vi "运维调试_氨氮.vi"() -> ()   [LabVIEW 2016, in "斯坦道氨氮.lvlib"]
uses:
  <vilib>/Utility/miscctls.llb/LVPointTypeDef.ctl
  <vilib>/Utility/config.llb/NI_LVConfig.lvlib
  <vilib>/ptbypt/NI_PtbyPt.lvlib
panel:
  in  "量程参数读取":T1
  in  "模块启用":bool
  in  "串口设置":bool
  in  "公式一键写入":bool
  in  "流程文件路径":path=path "C:/Users/Hsiao/Documents/斯坦道流程文件/流程.xml"
  in  "曲线模型":cluster{"X^2":dbl, "X":dbl, "B":dbl}(xcontrol)
  in  "质控参数设置":bool
  out "字符串":string
  in  "氨氮自动测试量程配置":T2
  out "ADC":sgl
  out "温度2":sgl
  out "温度1":sgl
  out "固件版本号":string
  in  "数组":string[](array[string])
  in  "备用系数写入":bool
  in  "备用系数读取":bool
  in  "参数下拉列表":enum16{"氨氮", "总磷"}(ring)
  in  "量程下拉列表":enum16{"低量程", "高量程"}(ring)
  in  "测量模式下拉列表":enum16{"水样测量", "空白核查", "跨度核查", "标样核查", "加标回收"}(ring)
  in  "公式":cluster{"X^2":dbl, "X":dbl, "b":dbl}
  in  "写公式":bool
  in  "读公式":bool
  in  "返回":bool
  in  "设置":bool
  out "序列号":string="序列号"
  out "氨氮测量数据":T3(xcontrol)
  out "集成报警信息":string
  out "定时启动":bool
  out "总磷总氮运行状态":T4(xcontrol)
  in  "停止":bool
  in  "手动启动":bool
  in  "单步测试":bool
  in  "总磷氨氮调试":u16[](xcontrol)
  out "F3":sgl format="%#.6f"
  out "F2":sgl format="%#.6f"
  out "F1":sgl format="%#.6f"
  out "F0":sgl format="%#.6f"
  out "多列列表框":i32(listbox)
  # "参数设置"
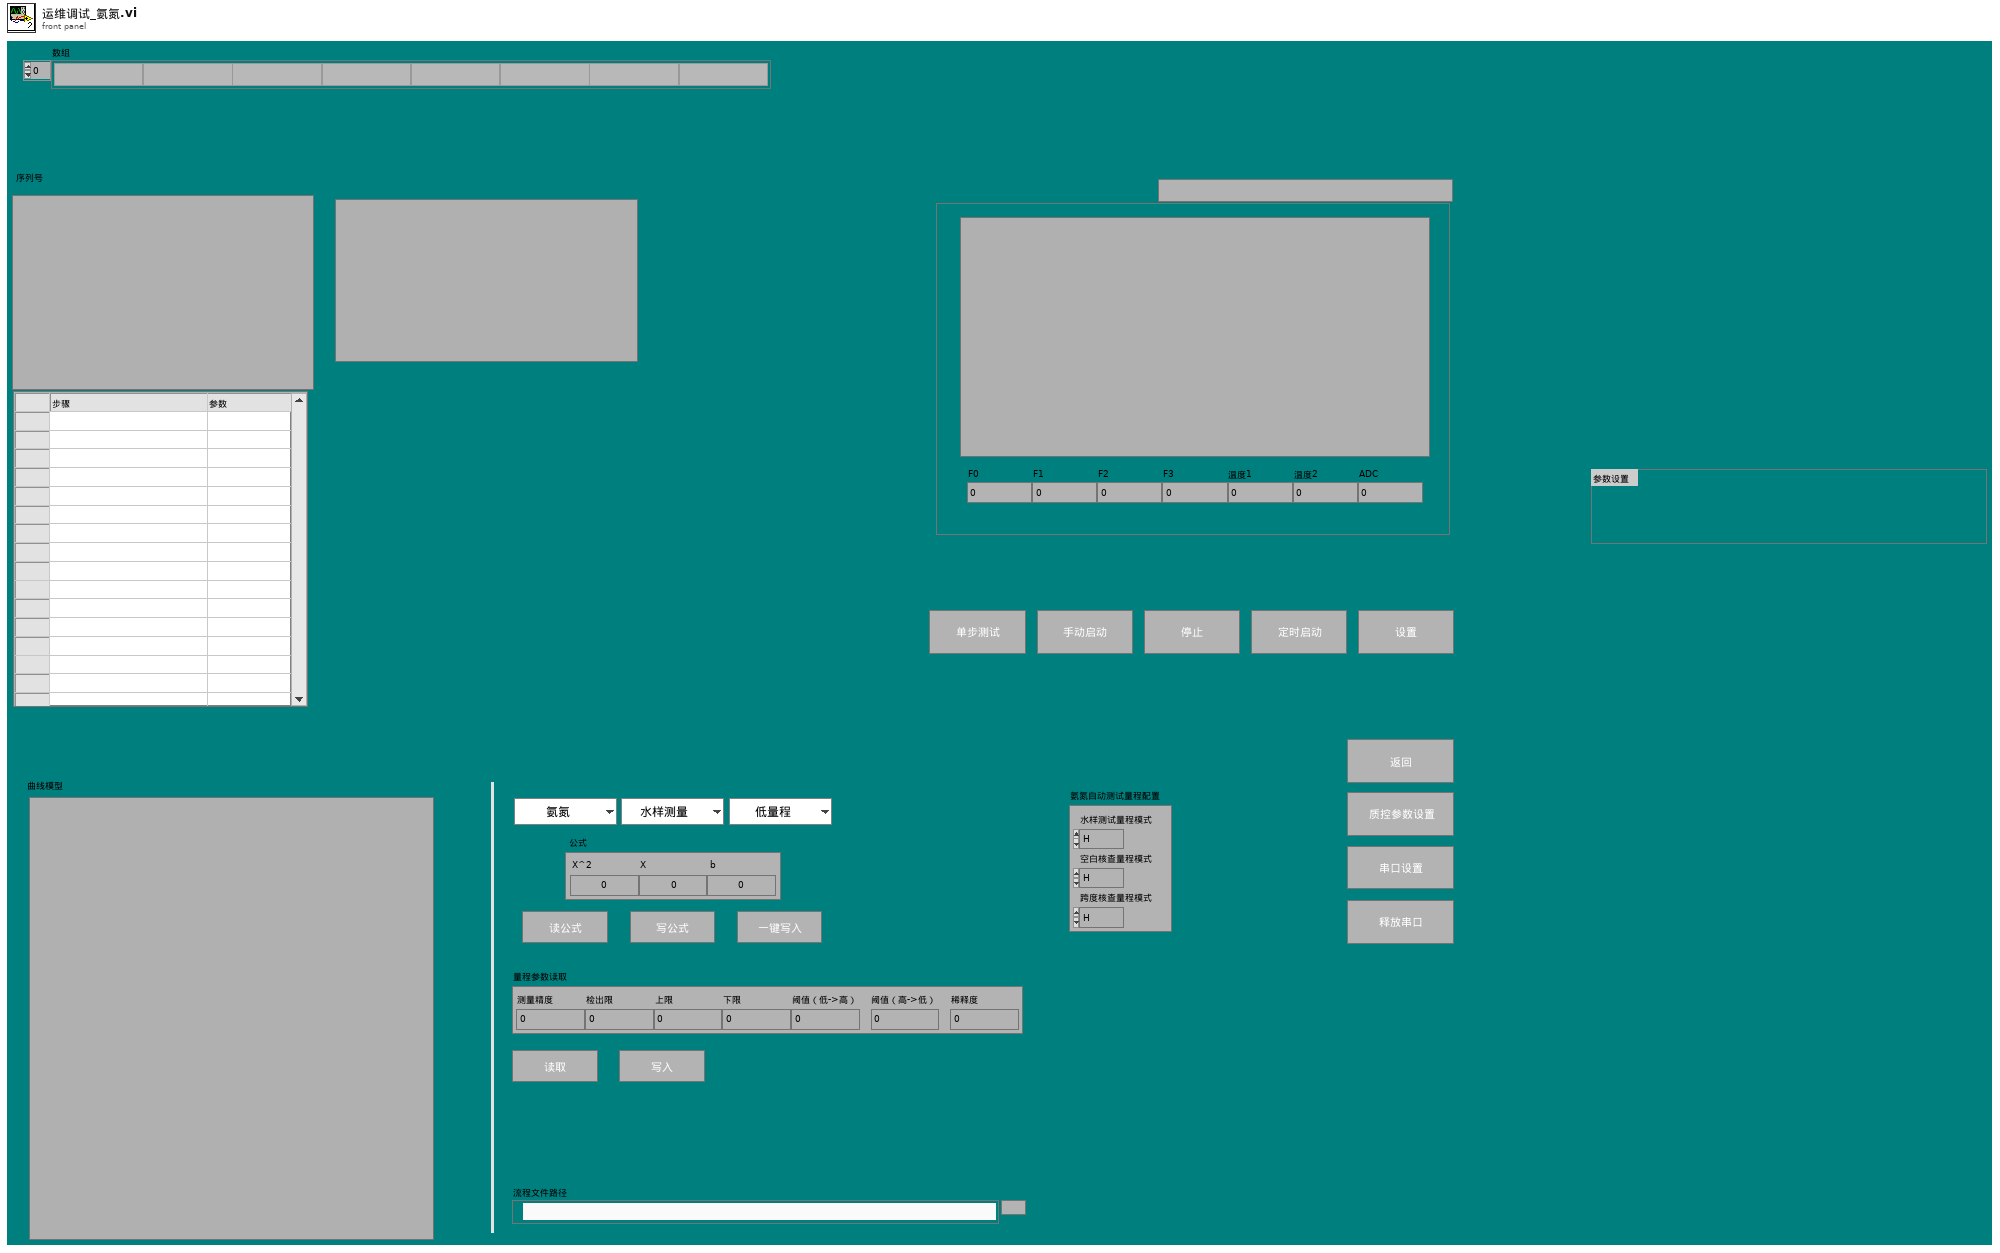
[diagram p1: front panel]
types:
  T1 = cluster{"测量精度":u16, "检出限":dbl, "上限":dbl, "下限":dbl, "阈值（低->高）":dbl, "阈值（高->低）":dbl, "稀释度":dbl}
  T2 = cluster{"水样测试量程模式":enum16{"H", "L", "AUTO"}, "空白核查量程模式":enum16{"H", "L", "AUTO"}, "跨度核查量程模式":enum16{"H", "L", "AUTO"}}
  T3 = cluster{"flowid":u16, "测量精度":u16, "测量数据区":cluster{"因子编码":u32, "单位":u16, "标样参考值":sgl, "水样数据时间":timestamp, "水样实测值":sgl, "水样数据标识":string, "标样数据时间":timestamp, "标样实测值":sgl, "标样数据标识":string, "空白数据时间":timestamp, "空白实测值":sgl, "空白数据标识":string, "零点核查数据时间":timestamp, "零点核查实测值":sgl, "零点核查数据标识":string, "跨度核查数据时间":timestamp, "跨度核查实测值":sgl, "跨度核查数据标识":string, "加标回收数据时间":timestamp, "加标回收实测值":sgl, "加标回收数据标识":string, "平行样数据时间":timestamp, "平行样实测值":sgl, "平行样数据标识":string, "F0":sgl, "F1":sgl, "F2":sgl, "F3":sgl, "F4":sgl, "F5":sgl, "F6":sgl, "F7":sgl, "温度":sgl, "湿度":sgl, "X值":sgl}}
  T4 = cluster{"系统时间":timestamp, "工作状态":enum16{"空闲", "水样测试", "标样核查", "零点核查", "跨度核查", "空白测试", "平行样测试", "加标回收", "空白校准", "标样校准", "初始化（清洗）"}, "测量模式":enum16{"待机", "连续模式", "周期模式", "定点模式", "受控模式", "手动模式"}, "告警代码":enum16{"无告警", "缺试剂告警", "缺水样告警", "缺蒸馏水告警", "缺标液告警", "仪表漏液告警", "标定异常告警", "超量程告警", "加热异常", "低试剂预警", "超上限告警", "超下限告警", "仪表内部其他异常", "滴定异常告警", "电极异常告警", "量程切换告警", "参数设置告警", "PH电极电位异常", "电导率电极异常", "浊度光度异常", "溶解氧电极异常", "溶解氧光强异常", "温度异常告警", "PH异常告警", "溶解氧异常告警", "电导率异常告警", "浊度异常告警", "叶绿素异常告警", "藻密度异常告警", "蓝绿藻异常告警", "ORP异常告警", "氨氮异常告警", "清洁刷异常告警", "SD卡异常告警", "蓝牙异常告警", "Wifi异常告警", "流程异常告警"}, "故障代码":enum16{"无故障", "电机故障", "温度故障", "通讯故障", "滴定故障"}, "日志代码":u16, "软件版本":u16, "F0":sgl, "F1":sgl, "F2":sgl, "F3":sgl, "T":sgl, "H":sgl, "id":u16, "flowid":u16, "量程":u16, "总磷控温温度1":sgl, "营养盐控温温度2":sgl, "ADC":sgl}
  T5 = cluster{"站号":u16, "量程切换":enum32{"H", "L", "AUTO"}, "控制命令":enum16{"启动测量", "标样核查", "零点核查", "跨度核查", "空白测试", "平行样测试", "加标回收", "空白校准", "标样校准", "初始化（清洗）", "停止测试", "仪器重启", "校时", "模式设置", "测量间隔设置"}, "模式设置":enum16{"待机", "连续模式", "周期模式", "定点模式", "受控模式", "手动模式"}, "测量间隔":u16}
  T6 = enum16{"启动测量", "标样核查", "零点核查", "跨度核查", "空白测试", "平行样测试", "加标回收", "空白校准", "标样校准", "初始化（清洗）", "停止测试", "仪器重启", "校时", "模式设置", "测量间隔设置"}
  T7 = cluster{"仪器测试类型":enum16{"水样测试", "标样核查", "空白测试", "跨度核查"}, "周期设置类型":enum16{"定点启动", "间隔启动"}, "定时功能启用":bool, "定时间隔":dbl, "24H周期设置":bool[]}
  T8 = enum32{"Bad", "Idle", "Run top level", "Running"}
  T9 = typedef "LVDateTimeRec.ctl" = cluster{"秒数的小数部分":dbl, "秒":i32, "分":i32, "时":i32, "日":i32, "月":i32, "年":i32, "天数（周）":i32, "天数（年）":i32, "DST":i32}
  T10 = typedef "LVPointTypeDef.ctl" = cluster{"Horizontal":i16, "Vertical":i16}
  T11 = cluster{"因子编码":u32, "单位":u16, "标样参考值":sgl, "水样数据时间":timestamp, "水样实测值":sgl, "水样数据标识":string, "标样数据时间":timestamp, "标样实测值":sgl, "标样数据标识":string, "空白数据时间":timestamp, "空白实测值":sgl, "空白数据标识":string, "零点核查数据时间":timestamp, "零点核查实测值":sgl, "零点核查数据标识":string, "跨度核查数据时间":timestamp, "跨度核查实测值":sgl, "跨度核查数据标识":string, "加标回收数据时间":timestamp, "加标回收实测值":sgl, "加标回收数据标识":string, "平行样数据时间":timestamp, "平行样实测值":sgl, "平行样数据标识":string, "F0":sgl, "F1":sgl, "F2":sgl, "F3":sgl, "F4":sgl, "F5":sgl, "F6":sgl, "F7":sgl, "T":sgl, "H":sgl, "X":sgl}
  T12 = enum16{"空闲", "水样测试", "标样核查", "零点核查", "跨度核查", "空白测试", "平行样测试", "加标回收", "空白校准", "标样校准", "初始化（清洗）"}
  T13 = typedef "NI_LVConfig.lvlib/Config Data RefNum.ctl" = refnum<k1>
  T14 = cluster{"启动模式":enum16{"跨度核查", "水样测量", "空白核查", "标样核查", "加标回收"}, "启动参数":u16, "量程":enum16{"低量程", "高量程"}}
  T15 = cluster{"时间标识":timestamp, "设备":string, "日志信息":string, "流程参数":string}
  T16 = cluster{"时间标识":timestamp, "设备":string, "日志信息":string}
  T17 = enum16{"无告警", "缺试剂告警", "缺水样告警", "缺蒸馏水告警", "缺标液告警", "仪表漏液告警", "标定异常告警", "超量程告警", "加热异常", "低试剂预警", "超上限告警", "超下限告警", "仪表内部其他异常", "滴定异常告警", "电极异常告警", "量程切换告警", "参数设置告警", "PH电极电位异常", "电导率电极异常", "浊度光度异常", "溶解氧电极异常", "溶解氧光强异常", "温度异常告警", "PH异常告警", "溶解氧异常告警", "电导率异常告警", "浊度异常告警", "叶绿素异常告警", "藻密度异常告警", "蓝绿藻异常告警", "ORP异常告警", "氨氮异常告警", "清洁刷异常告警", "SD卡异常告警", "蓝牙异常告警", "Wifi异常告警", "流程异常告警"}
  T18 = typedef "LVRowAndColumnUnsignedTypeDef.ctl" = cluster{"Row":u32, "Column":u32}
  T19 = cluster{"跨度值":dbl, "零点标准液浓度":dbl, "跨度标准液浓度":dbl, "标准液标准浓度":dbl}
  T20 = cluster{"确定":bool, "跨度值":dbl, "零点标准液浓度":dbl, "跨度标准液浓度":dbl, "标准液标准浓度":dbl}
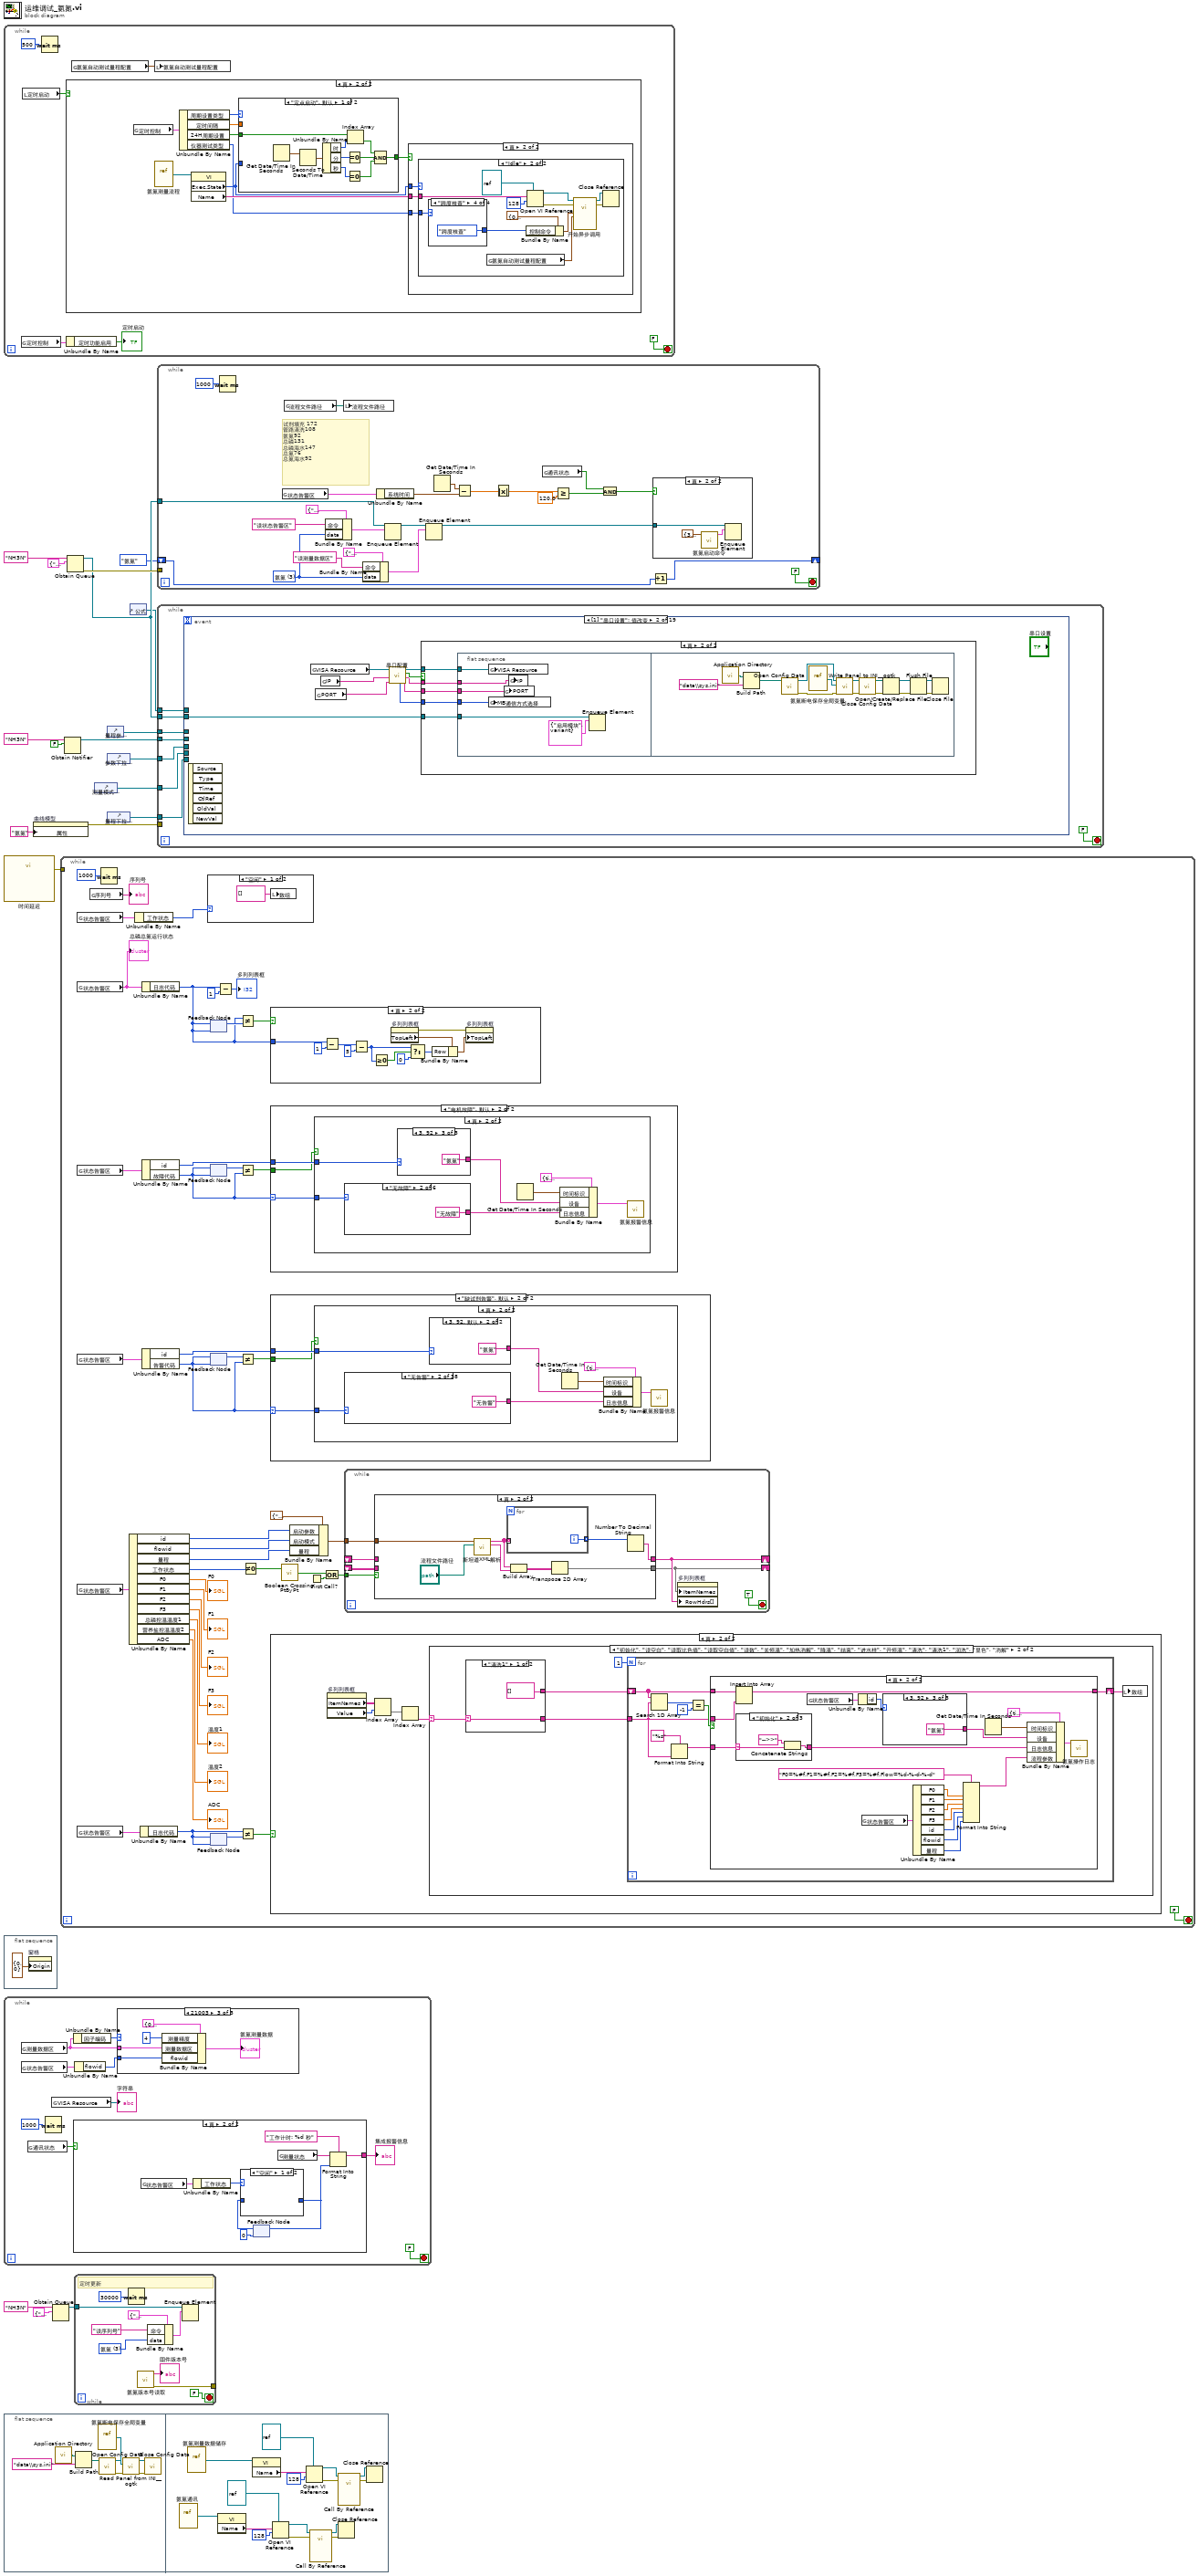
[diagram p0: block diagram]
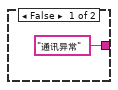
[diagram p2: hidden frame]
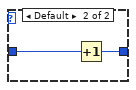
[diagram p3: hidden frame]
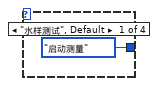
[diagram p9: hidden frame]
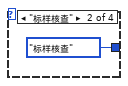
[diagram p10: hidden frame]
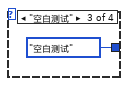
[diagram p11: hidden frame]
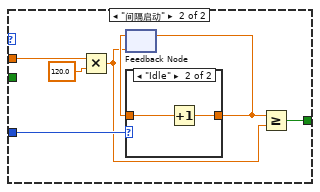
[diagram p12: hidden frame]
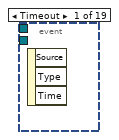
[diagram p14: hidden frame]
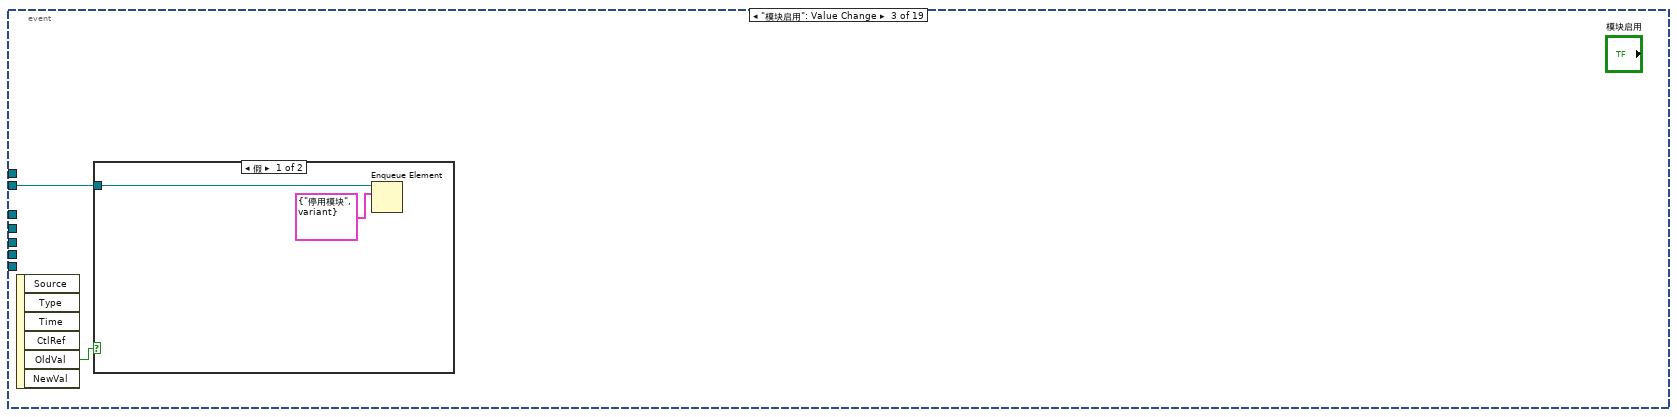
[diagram p16: hidden frame]
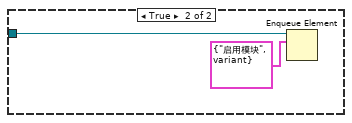
[diagram p17: hidden frame]
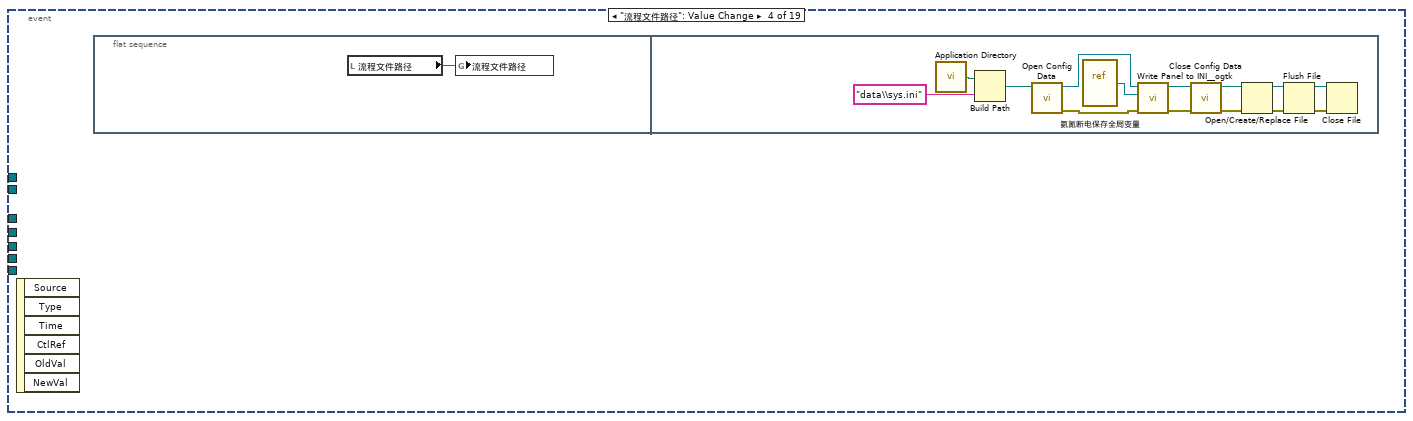
[diagram p18: hidden frame]
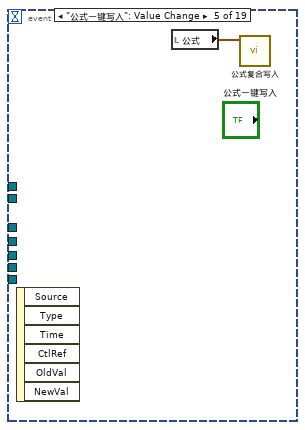
[diagram p19: hidden frame]
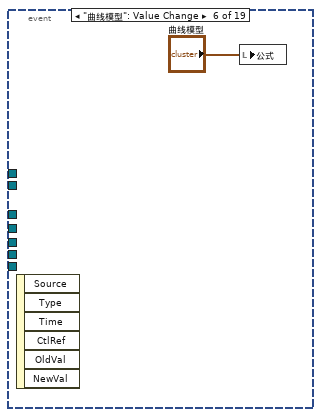
[diagram p20: hidden frame]
diagram:
  n1 = while {
    stop <- FALSE stop-if-true
    n2 = global read "氨氮断电保存全局变量.vi" "定时控制"() -> (w22:T7)
    n3 = local read "定时启动"() -> (w23:bool)
    n4 = Wait (ms)(milliseconds to wait=u32 500 ("等待时间（毫秒）")) -> ()  [unwired: 1 out]
    n5 = case shown="真" w23 {
      frame False {
      }
      frame True {
        n6 = global read "氨氮断电保存全局变量.vi" "定时控制"() -> (w34:T7)
        n7 = vi-ref "氨氮测量流程.vi"() -> (w30:refnum<vi>)
        n8 = Unbundle By Name(w34) -> ("周期设置类型"=w33:enum16{"定点启动", "间隔启动"}, "定时间隔"=w32:dbl, "24H周期设置"=w31:bool[], "仪器测试类型"=w27:enum16{"水样测试", "标样核查", "空白测试", "跨度核查"})
        n9 = property class="VI"(reference=w30) -> ("Exec.State"=w26:T8, "Name"=w29:string)  [unwired: 1 in, 2 out]
        n10 = case shown="\"定点启动\", 默认" w33 {
          tunnel: w32 -> [_ w67]
          tunnel: w31 -> [w63 _]
          tunnel: w26 -> [_ w70]
          tunnel: [w62 w65] -> w28
          frame "定点启动", Default {
            n11 = Get Date/Time In Seconds() -> (seconds since 1Jan1904=w61:timestamp)
            n12 = Seconds To Date/Time(time stamp (now)=w61) -> (date time rec=w60:T9)  [unwired: 1 in]
            n13 = Unbundle By Name(w60) -> ("时"=w59:i32, "分"=w57:i32, "秒"=w58:i32)
            n14 = Equal To 0?(x=w57) -> (x = 0?=w55:bool)
            n15 = Equal To 0?(x=w58) -> (x = 0?=w54:bool)
            n16 = Index Array(array=w63, index=w59) -> (element=w56:bool)
            n17 = Compound Arithmetic op=AND ("复合运算")(w56, w55, w54) -> (w62:bool)
          }
          frame "间隔启动" {
            n18 = Multiply(x=w67, y=120.0) -> (x*y=w64:dbl)
            n19 = feedback #1(w64) -> (w69:dbl)
            n20 = case shown="\"Idle\"" w70 {
              tunnel: w69 -> [_ w72]
              tunnel: [_ w71] -> w68
              frame "Bad", Default {
              }
              frame "Idle" {
                n21 = Increment(x=w72) -> (x+1=w71:dbl)
              }
            }
            n22 = feedback-in #1(w68) -> ()
            n23 = Greater Or Equal?(x=w68, y=w64) -> (x >= y?=w65:bool)
          }
        }
        n24 = case shown="真" w28 {
          tunnel: w29 -> [_ w37]
          tunnel: w27 -> [_ w36]
          tunnel: w26 -> [_ w35]
          frame False {
          }
          frame True {
            n25 = case shown="\"Idle\"" w35 {
              tunnel: w37 -> [_ w44]
              tunnel: w36 -> [_ w40]
              frame "Bad", Default {
              }
              frame "Idle" {
                n26 = case shown="\"跨度核查\"" w40 {
                  tunnel: [T6."启动测量" ("控制命令") T6."标样核查" ("控制命令") T6."空白测试" ("控制命令") T6."跨度核查" ("控制命令")] -> w39
                  frame "水样测试", Default {
                  }
                  frame "标样核查" {
                  }
                  frame "空白测试" {
                  }
                  frame "跨度核查" {
                  }
                }
                n27 = global read "氨氮断电保存全局变量.vi" "氨氮自动测试量程配置"() -> (w38:T2)
                n28 = Bundle By Name(cluster=T5 {"站号"=0, "量程切换"=enum."H", "控制命令"=enum."启动测量", "模式设置"=enum."待机", "测量间隔"=0} ("参数"), "控制命令"=w39) -> (w41:T5)
                n29 = Open VI Reference(type specifier VI Refnum (for type only)=refnum<vi> refnum, vi path=w44, options=128 ("选项")) -> (vi reference=w45:refnum<vi>, error out=w46:errorcluster)  [unwired: 3 in]
                n30 = call-by-ref "开始异步调用"(reference=w45, error in=w46, "量程模式"=w38, "参数"=w41) -> (reference out=w47:refnum<vi>, error out=w48:errorcluster)  [unwired: 10 in]
                n31 = Close Reference(reference=w47, error in (no error)=w48) -> ()  [unwired: 1 out]
              }
            }
          }
        }
      }
    }
    n32 = Unbundle By Name(w22) -> ("定时功能启用"=→"定时启动":bool)
    n33 = global read "氨氮断电保存全局变量.vi" "氨氮自动测试量程配置"() -> (w20:T2)
    n34 = local write "氨氮自动测试量程配置"(w20) -> ()
  }
  n35 = call "时间延迟"() -> ("error out"=w10:errorcluster)  [unwired: 11 in]
  n36 = flat-sequence {
    frame #0 {
      n37 = property on="窗格" class="Pane"("Origin"=T10 {"Horizontal"=0, "Vertical"=0} ("原点")) -> ()  [unwired: 2 in, 2 out]
    }
  }
  n38 = while {
    stop <- FALSE stop-if-true
    n39 = global read "VAR氨氮全局变量.vi" "测量数据区"() -> (w80:T11)
    n40 = global read "VAR氨氮全局变量.vi" "状态告警区"() -> (w76:T4)
    n41 = global read "VAR氨氮全局变量.vi" "通讯状态"() -> (w78:bool)
    n42 = Wait (ms)(milliseconds to wait=u32 1000 ("等待时间（毫秒）")) -> ()  [unwired: 1 out]
    n43 = global read "氨氮断电保存全局变量.vi" "VISA Resource"() -> (→"字符串":refnum<visa-resource-name>)
    n44 = Unbundle By Name(w80) -> ("因子编码"=w79:u32)
    n45 = case shown="真" w78 {
      tunnel: ["通讯异常" ("集成报警信息") w85] -> w77
      frame False {
      }
      frame True {
        n46 = global read "VAR氨氮全局变量.vi" "状态告警区"() -> (w91:T4)
        n47 = Unbundle By Name(w91) -> ("工作状态"=w90:T12)
        n48 = feedback #2(0) -> (w88:i32)
        n49 = case shown="\"空闲\"" w90 {
          tunnel: w88 -> [_ w93]
          tunnel: [_ w92] -> w86
          frame "空闲" {
          }
          frame Default {
            n50 = Increment(x=w93) -> (x+1=w92:i32)
          }
        }
        n51 = feedback-in #2(w86) -> ()
        n52 = global read "VAR氨氮全局变量.vi" "测量状态"() -> (w84:string)
        n53 = Format Into String(format string="工作计时: %d 秒" ("格式字符串"), initial string=w84, w86) -> (resulting string=w85:string)  [unwired: 1 in, 1 out]
      }
    }
    "集成报警信息" <- w77
    n54 = Unbundle By Name(w76) -> ("flowid"=w75:u16)
    n55 = case shown="21003" w79 {
      tunnel: w80 -> [_ _ w98]
      tunnel: w75 -> [_ _ w96]
      frame Default {
      }
      frame 21011 {
      }
      frame 21003 {
        n56 = Bundle By Name(cluster=T3 {"flowid"=0, "测量精度"=0, "测量数据区"={"因子编码"=0, "单位"=0, "标样参考值"=0.0, "水样数据时间"=timestamp(0 s since 1904-01-01), "水样实测值"=0.0, "水样数据标识"="", "标样数据时间"=timestamp(0 s since 1904-01-01), "标样实测值"=0.0, "标样数据标识"="", "空白数据时间"=timestamp(0 s since 1904-01-01), "空白实测值"=0.0, "空白数据标识"="", "零点核查数据时间"=timestamp(0 s since 1904-01-01), "零点核查实测值"=0.0, "零点核查数据标识"="", "跨度核查数据时间"=timestamp(0 s since 1904-01-01), "跨度核查实测值"=0.0, "跨度核查数据标识"="", "加标回收数据时间"=timestamp(0 s since 1904-01-01), "加标回收实测值"=0.0, "加标回收数据标识"="", "平行样数据时间"=timestamp(0 s since 1904-01-01), "平行样实测值"=0.0, "平行样数据标识"="", "F0"=0.0, "F1"=0.0, "F2"=0.0, "F3"=0.0, "F4"=0.0, "F5"=0.0, "F6"=0.0, "F7"=0.0, "温度"=0.0, "湿度"=0.0, "X值"=0.0}} ("氨氮测量数据"), "测量精度"=u16 4, "测量数据区"=w98, "flowid"=w96) -> (→"氨氮测量数据":T3)
      }
    }
  }
  n57 = flat-sequence {
    frame #0 {
      n58 = call <vilib>:"Application Directory.vi"() -> ("Application Directory"=w99:path)
      n59 = Build Path(base path=w99, name or relative path="data\\sys.ini" ("名称或相对路径")) -> (appended path=w101:path)
      n60 = vi-ref "氨氮断电保存全局变量.vi"() -> (w103:refnum<vi>)
      n61 = call <vilib>:"Open Config Data.vi"("configuration file path"=w101) -> ("error out"=w105:errorcluster, "refnum"=w102:T13)  [unwired: 8 in, 1 out]
      n62 = call <userlib>:"Read Panel from INI__ogtk.vi"("error in (no error)"=w105, "VI ref"=w103, "refnum"=w102) -> ("error out"=w106:errorcluster, "refnum out"=w104:T13)  [unwired: 7 in]
      n63 = call <vilib>:"Close Config Data.vi"("error in (no error)"=w106, "refnum"=w104) -> ()  [unwired: 8 in, 2 out]
    }
    frame #1 {
      n64 = vi-ref "氨氮通讯.vi"() -> (w122:refnum<vi>)
      n65 = vi-ref "氨氮测量数据储存.vi"() -> (w114:refnum<vi>)
      n66 = property class="VI"(reference=w122) -> ("Name"=w121:string)  [unwired: 1 in, 2 out]
      n67 = property class="VI"(reference=w114) -> ("Name"=w107:string)  [unwired: 1 in, 2 out]
      n68 = Open VI Reference(type specifier VI Refnum (for type only)=refnum<vi> refnum, vi path=w121, options=128 ("选项")) -> (vi reference=w119:refnum<vi>, error out=w117:errorcluster)  [unwired: 3 in]
      n69 = Open VI Reference(type specifier VI Refnum (for type only)=refnum<vi> refnum, vi path=w107, options=128 ("选项")) -> (vi reference=w109:refnum<vi>, error out=w111:errorcluster)  [unwired: 3 in]
      n70 = call-by-ref "?"(reference=w119, error in=w117) -> (reference out=w115:refnum<vi>, error out=w116:errorcluster)  [unwired: 12 in]
      n71 = call-by-ref "?"(reference=w109, error in=w111) -> (reference out=w113:refnum<vi>, error out=w112:errorcluster)  [unwired: 12 in]
      n72 = Close Reference(reference=w115, error in (no error)=w116) -> ()  [unwired: 1 out]
      n73 = Close Reference(reference=w113, error in (no error)=w112) -> ()  [unwired: 1 out]
    }
  }
  n74 = property on="曲线模型" class="氨氮曲线模型 (严格)"("属性"="氨氮" ("调用模块名称属性")) -> (error out=w3:errorcluster)  [unwired: 2 in, 1 out]
  n75 = Obtain Queue(name (unnamed)="NH3N" ("名称（未命名）"), element data type=cluster{"命令":string, "data":variant} {"命令"="", "data"=variant}) -> (queue out=w7:refnum<queue>)  [unwired: 3 in, 2 out]
  n76 = while {
    tunnel: w10 -> [_]
    stop <- FALSE stop-if-true
    n77 = global read "VAR氨氮全局变量.vi" "状态告警区"() -> (w138:T4)
    n78 = global read "VAR氨氮全局变量.vi" "状态告警区"() -> (w150:T4)
    "总磷总氮运行状态" <- w150
    n79 = global read "VAR氨氮全局变量.vi" "状态告警区"() -> (w143:T4)
    n80 = global read "VAR氨氮全局变量.vi" "状态告警区"() -> (w148:T4)
    n81 = global read "VAR氨氮全局变量.vi" "状态告警区"() -> (w158:T4)
    n82 = global read "VAR氨氮全局变量.vi" "状态告警区"() -> (w135:T4)
    n83 = global read "VAR氨氮全局变量.vi" "序列号"() -> (→"序列号":string)
    n84 = Wait (ms)(milliseconds to wait=u32 1000 ("等待时间（毫秒）")) -> ()  [unwired: 1 out]
    n85 = Unbundle By Name(w158) -> ("id"=w155:u16, "flowid"=w157:u16, "量程"=w156:u16, "工作状态"=w124:T12, "F0"=→"F0":sgl, "F1"=→"F1":sgl, "F2"=→"F2":sgl, "F3"=→"F3":sgl, "总磷控温温度1"=→"温度1":sgl, "营养盐控温温度2"=→"温度2":sgl, "ADC"=→"ADC":sgl)
    n86 = Unbundle By Name(w138) -> ("工作状态"=w137:T12)
    n87 = Unbundle By Name(w135) -> ("日志代码"=w134:u16)
    n88 = Unbundle By Name(w150) -> ("日志代码"=w128:u16)
    n89 = Unbundle By Name(w143) -> ("id"=w142:u16, "故障代码"=w139:enum16{"无故障", "电机故障", "温度故障", "通讯故障", "滴定故障"})
    n90 = Unbundle By Name(w148) -> ("id"=w147:u16, "告警代码"=w144:T17)
    n91 = case shown="\"空闲\"" w137 {
      frame "空闲" {
        n92 = local write "数组"(string[] [] ("数组")) -> ()
      }
      frame "水样测试", Default {
      }
    }
    n93 = feedback-in #3(w128) -> ()
    n94 = feedback #3(w128) -> (w163:u16)
    n95 = feedback #4(w139) -> (w140:enum16{"无故障", "电机故障", "温度故障", "通讯故障", "滴定故障"})
    n96 = feedback-in #4(w139) -> ()
    n97 = feedback #5(w144) -> (w145:T17)
    n98 = feedback-in #5(w144) -> ()
    n99 = feedback #6(w134) -> (w136:u16)
    n100 = feedback-in #6(w134) -> ()
    n101 = Subtract(x=w128, y=1) -> (x-y=→"多列列表框":i32)
    n102 = Not Equal?(x=w128, y=w163) -> (x != y?=w162:bool)
    n103 = Not Equal?(x=w140, y=w139) -> (x != y?=w141:bool)
    n104 = Not Equal?(x=w145, y=w144) -> (x != y?=w146:bool)
    n105 = Not Equal?(x=w134, y=w136) -> (x != y?=w133:bool)
    n106 = Not Equal To 0?(x=w124) -> (x != 0?=w160:bool)
    n107 = case shown="真" w162 {
      tunnel: w128 -> [_ w313]
      frame False {
      }
      frame True {
        n108 = Subtract(x=w313, y=1) -> (x-y=w311:i32)
        n109 = Subtract(x=w311, y=5) -> (x-y=w315:i32)
        n110 = Greater Or Equal To 0?(x=w315) -> (x >= 0?=w314:bool)
        n111 = property on="多列列表框" class="MCListbox (严格)"() -> (error out=w319:errorcluster, "TopLeft"=w320:T18)  [unwired: 2 in, 1 out]
        n112 = Select(t=w315, s=w314, f=0) -> (s? t:f=w316:i32)
        n113 = Bundle By Name(cluster=w320, "Row"=w316) -> (w321:T18)
        n114 = property on="多列列表框" class="MCListbox (严格)"(error in=w319, "TopLeft"=w321) -> ()  [unwired: 1 in, 2 out]
      }
    }
    n115 = case shown="\"电机故障\", 默认" w139 {
      selector: w139 -> [_ w220]
      tunnel: w142 -> [_ w221]
      tunnel: w141 -> [_ w219]
      frame "无故障" {
      }
      frame "电机故障", Default {
        n116 = case shown="真" w219 {
          tunnel: w221 -> [_ w228]
          tunnel: w220 -> [_ w223]
          frame False {
          }
          frame True {
            n117 = case shown="\"无故障\"" w223 {
              selector: w223 -> [w230 _ _ _ _ _]
              tunnel: [w229 "无故障" "电机故障" "温度故障" "通讯故障" "滴定故障"] -> w222
              frame Default {
                n118 = Format Into String(format string="%d" ("格式字符串"), initial string="未知" ("工作状态"), w230) -> (resulting string=w229:string)  [unwired: 1 in, 1 out]
              }
              frame "无故障" {
              }
              frame "电机故障" {
              }
              frame "温度故障" {
              }
              frame "通讯故障" {
              }
              frame "滴定故障" {
              }
            }
            n119 = case shown="3, 92" w228 {
              tunnel: [_ "总磷" ("table输入") "氨氮" ("table输入")] -> w224
              frame Default {
              }
              frame 1, 131 {
              }
              frame 3, 92 {
              }
            }
            n120 = Get Date/Time In Seconds() -> (seconds since 1Jan1904=w225:timestamp)
            n121 = Bundle By Name(cluster=T16 {"时间标识"=timestamp(0 s since 1904-01-01), "设备"="", "日志信息"=""} ("data in"), "时间标识"=w225, "设备"=w224, "日志信息"=w222) -> (w226:T16)
            n122 = call "氨氮报警信息.vi"("data in"=w226) -> ()  [unwired: 11 in]
          }
        }
      }
    }
    n123 = case shown="\"缺试剂告警\", 默认" w144 {
      selector: w144 -> [_ w241]
      tunnel: w147 -> [_ w242]
      tunnel: w146 -> [_ w240]
      frame "无告警" {
      }
      frame "缺试剂告警", Default {
        n124 = case shown="真" w240 {
          tunnel: w242 -> [_ w249]
          tunnel: w241 -> [_ w243]
          frame False {
          }
          frame True {
            n125 = case shown="\"无告警\"" w243 {
              selector: w243 -> [w251 _ _ _ _ _ _ _ _ _ _ _ _ _ _ _ _ _ _ _ _ _ _ _ _ _ _ _ _ _ _ _ _ _ _ _ _ _]
              tunnel: [w250 "无告警" "缺试剂告警" "缺水样告警" "缺蒸馏水告警" "缺标液告警" "仪表漏液告警" "标定异常告警" "超量程告警" "加热异常" "低试剂预警" "超上限告警" "超下限告警" "仪表内部其他异常" "滴定异常告警" "电极异常告警" "量程切换告警" "参数设置告警" "PH电极电位异常" "电导率电极异常" "浊度光度异常" "溶解氧电极异常" "溶解氧光强异常" "温度异常告警" "PH异常告警" "溶解氧异常告警" "电导率异常告警" "浊度异常告警" "叶绿素异常告警" "藻密度异常告警" "蓝绿藻异常告警" "ORP异常告警" "氨氮异常告警" "清洁刷异常告警" "SD卡异常告警" "蓝牙异常告警" "WiFi异常告警" "流程异常告警"] -> w244
              frame Default {
                n126 = Format Into String(format string="%d" ("格式字符串"), initial string="未知" ("工作状态"), w251) -> (resulting string=w250:string)  [unwired: 1 in, 1 out]
              }
              frame "无告警" {
              }
              frame "缺试剂告警" {
              }
              frame "缺水样告警" {
              }
              frame "缺蒸馏水告警" {
              }
              frame "缺标液告警" {
              }
              frame "仪表漏液告警" {
              }
              frame "标定异常告警" {
              }
              frame "超量程告警" {
              }
              frame "加热异常" {
              }
              frame "低试剂预警" {
              }
              frame "超上限告警" {
              }
              frame "超下限告警" {
              }
              frame "仪表内部其他异常" {
              }
              frame "滴定异常告警" {
              }
              frame "电极异常告警" {
              }
              frame "量程切换告警" {
              }
              frame "参数设置告警" {
              }
              frame "PH电极电位异常" {
              }
              frame "电导率电极异常" {
              }
              frame "浊度光度异常" {
              }
              frame "溶解氧电极异常" {
              }
              frame "溶解氧光强异常" {
              }
              frame "温度异常告警" {
              }
              frame "PH异常告警" {
              }
              frame "溶解氧异常告警" {
              }
              frame "电导率异常告警" {
              }
              frame "浊度异常告警" {
              }
              frame "叶绿素异常告警" {
              }
              frame "藻密度异常告警" {
              }
              frame "蓝绿藻异常告警" {
              }
              frame "ORP异常告警" {
              }
              frame "氨氮异常告警" {
              }
              frame "清洁刷异常告警" {
              }
              frame "SD卡异常告警" {
              }
              frame "蓝牙异常告警" {
              }
              frame "Wifi异常告警" {
              }
              frame "流程异常告警" {
              }
            }
            n127 = case shown="3, 92, 默认" w249 {
              tunnel: ["总磷" ("table输入") "氨氮" ("table输入")] -> w245
              frame 1, 131 {
              }
              frame 3, 92, Default {
              }
            }
            n128 = Get Date/Time In Seconds() -> (seconds since 1Jan1904=w246:timestamp)
            n129 = Bundle By Name(cluster=T16 {"时间标识"=timestamp(0 s since 1904-01-01), "设备"="", "日志信息"=""} ("data in"), "时间标识"=w246, "设备"=w245, "日志信息"=w244) -> (w247:T16)
            n130 = call "氨氮报警信息.vi"("data in"=w247) -> ()  [unwired: 11 in]
          }
        }
      }
    }
    n131 = case shown="真" w133 {
      frame False {
      }
      frame True {
        n132 = property on="多列列表框" class="MCListbox (严格)"() -> ("ItemNames"=w169:string[][], "Value"=w170:i32)  [unwired: 2 in, 2 out]
        n133 = Index Array(array=w169, index (row)=w170) -> (element=w168:string[])  [unwired: 1 in]
        n134 = Index Array(array=w168) -> (element=w167:string)  [unwired: 1 in]
        n135 = case shown="\"初始化\", \"读空白\", \"读取比色值\", \"读取空白值\", \"读数\", \"关恒温\", \"加热消解\", \"降温\", \"结束\", \"进水样\", \"开恒温\", \"清洗\", \"清洗1\", \"润洗\", \"显色\", \"消解\"" w167 {
          selector: w167 -> [_ w173]
          frame Default {
          }
          frame "初始化", "读空白", "读取比色值", "读取空白值", "读数", "关恒温", "加热消解", "降温", "结束", "进水样", "开恒温", "清洗", "清洗1", "润洗", "显色", "消解" {
            n136 = case shown="\"清洗1\"" w173 {
              selector: w173 -> [w177 w179]
              tunnel: [w177 w179] -> w172
              tunnel: [string[] [] ("数组") "数组"] -> w171
              frame "清洗1" {
              }
              frame Default {
              }
            }
            n137 = for {
              N: 1 -> [_]
              tunnel: w172 -> [w181]
              shift-right: [w180] -> w174
              shift-left: w171 -> [w182]
              n138 = Search 1D Array(1D array=w182, element=w181) -> (index of element=w185:i32)  [unwired: 1 in]
              n139 = Format Into String(format string="%s" ("格式字符串"), w181) -> (resulting string=w186:string)  [unwired: 2 in, 1 out]
              n140 = Equal?(x=w185, y=-1) -> (x = y?=w183:bool)
              n141 = case shown="真" w183 {
                tunnel: w186 -> [_ w190]
                tunnel: w182 -> [w188 w194]
                tunnel: w181 -> [_ w193]
                tunnel: [w188 w192] -> w180
                frame False {
                }
                frame True {
                  n142 = Insert Into Array(array=w194, new element=w193) -> (w192:string[])  [unwired: 1 in]
                  n143 = case shown="\"初始化\"" w190 {
                    selector: w190 -> [w210 w213 w216]
                    tunnel: [w210 w212 w215] -> w189
                    frame Default {
                    }
                    frame "初始化" {
                      n144 = Concatenate Strings("-->>" ("字符串"), w213) -> (w212:string)
                    }
                    frame "结束" {
                      n145 = Concatenate Strings("-->>" ("字符串"), w216) -> (w215:string)
                    }
                  }
                  n146 = global read "VAR氨氮全局变量.vi" "状态告警区"() -> (w209:T4)
                  n147 = Unbundle By Name(w209) -> ("id"=w208:u16)
                  n148 = global read "VAR氨氮全局变量.vi" "状态告警区"() -> (w204:T4)
                  n149 = case shown="3, 92" w208 {
                    tunnel: [_ "总磷" ("table输入") "氨氮" ("table输入")] -> w206
                    frame Default {
                    }
                    frame 1, 131 {
                    }
                    frame 3, 92 {
                    }
                  }
                  n150 = Unbundle By Name(w204) -> ("F0"=w201:sgl, "F1"=w200:sgl, "F2"=w199:sgl, "F3"=w198:sgl, "id"=w197:u16, "flowid"=w196:u16, "量程"=w195:u16)
                  n151 = Format Into String(format string="F0=%#f,F1=%#f,F2=%#f,F3=%#f,Flow=%d-%-d-%-d" ("格式字符串"), w201, w200, w199, w198, w197, w196, w195) -> (resulting string=w202:string)  [unwired: 2 in, 1 out]
                  n152 = Get Date/Time In Seconds() -> (seconds since 1Jan1904=w205:timestamp)
                  n153 = Bundle By Name(cluster=T15 {"时间标识"=timestamp(0 s since 1904-01-01), "设备"="", "日志信息"="", "流程参数"=""} ("data in"), "时间标识"=w205, "设备"=w206, "日志信息"=w189, "流程参数"=w202) -> (w207:T15)
                  n154 = call "氨氮操作日志.vi"("data in"=w207) -> ()  [unwired: 11 in]
                }
              }
            }
            n155 = local write "数组"(w174) -> ()
          }
        }
      }
    }
    n156 = call <vilib>:"Boolean Crossing PtByPt.vi"("input"=w160) -> ("crossing"=w123:bool)  [unwired: 2 in]
    n157 = Bundle By Name(cluster=T14 {"启动模式"=enum."跨度核查", "启动参数"=1, "量程"=enum."低量程"} ("参数簇"), "启动参数"=w155, "启动模式"=w157, "量程"=w156) -> (w125:T14)
    n158 = First Call?() -> (First Call?: T/F=w161:bool)
    n159 = Or(x=w123, y=w161) -> (x .or. y?=w159:bool)
    n160 = while {
      tunnel: w159 -> [w299]
      tunnel: w125 -> [w298]
      shift-right: [w293] -> _
      shift-left: _ -> [w295]
      shift-right: [w294] -> _
      shift-left: _ -> [w296]
      stop <- TRUE stop-if-true
      n161 = case shown="真" w299 {
        tunnel: [w301 w309] -> w294
        tunnel: [w300 w308] -> w293
        tunnel: w298 -> [_ w303]
        tunnel: w296 -> [w301 _]
        tunnel: w295 -> [w300 _]
        frame False {
        }
        frame True {
          n162 = call "斯坦道XML解析.vi"("添加的路径"="流程文件路径", "参数簇"=w303) -> ("步骤时间"=w304:string[], "步骤名"=w306:string[])  [unwired: 8 in]
          n163 = for {
            tunnel: w306 -> [_] mode=indexing
            tunnel: [w310] -> w307 mode=indexing
            i -> [w310]
          }
          n164 = Build Array(w306, w304) -> (w305:string[][])
          n165 = Transpose 2D Array(2D array=w305) -> (transposed array=w308:string[][])
          n166 = Number To Decimal String(number=w307) -> (decimal integer string=w309:string[])  [unwired: 1 in]
        }
      }
      n167 = property on="多列列表框" class="MCListbox (严格)"("ItemNames"=w293, "RowHdrs[]"=w294) -> ()  [unwired: 2 in, 2 out]
    }
  }
  n168 = Obtain Notifier(name (unnamed)="NH3N" ("名称（未命名）"), notification data type=FALSE) -> (notifier out=w4:refnum<notifier>)  [unwired: 2 in, 2 out]
  n169 = Obtain Queue(name (unnamed)="NH3N" ("名称（未命名）"), element data type=cluster{"命令":string, "data":variant} {"命令"="", "data"=variant}) -> (queue out=w16:refnum<queue>, error out=w17:errorcluster)  [unwired: 3 in, 1 out]
  n170 = while {
    tunnel: w7 -> [w326]
    tunnel: [w323] -> _
    stop <- FALSE stop-if-true
    w327 = u16 3 items=["总磷"=1, "氨氮"=3] ("站号")
    # "定时更新"
    n171 = Wait (ms)(milliseconds to wait=u32 30000 ("等待时间（毫秒）")) -> ()  [unwired: 1 out]
    n172 = call "氨氮版本号读取.vi"() -> ("error out"=w323:errorcluster, "固件版本号"=→"固件版本号":string)  [unwired: 10 in]
    n173 = Bundle By Name(cluster=cluster{"命令":string, "data":variant} {"命令"="", "data"=variant} ("元素"), "命令"="读序列号", "data"=w327) -> (w325:cluster{"命令":string, "data":variant})
    n174 = Enqueue Element(queue=w326, element=w325) -> ()  [unwired: 2 in, 3 out]
  }
  n175 = control-ref of="测量模式下拉列表"() -> (w12:refnum<vi>)
  n176 = control-ref of="量程参数读取"() -> (w1:refnum<vi>)
  n177 = control-ref of="参数下拉列表"() -> (w13:refnum<vi>)
  n178 = control-ref of="量程下拉列表"() -> (w14:refnum<vi>)
  n179 = control-ref of="公式"() -> (w11:refnum<vi>)
  n180 = while {
    tunnel: w16 -> [w349]
    tunnel: w17 -> [_]
    shift-right: [w343] -> _
    shift-left: enum16{"氨氮", "总磷"}."氨氮" ("枚举") -> [w344]
    stop <- FALSE stop-if-true
    w342 = u16 3 items=["总磷"=1, "氨氮"=3] ("站号")
    # "试剂填充 172 \n管路清洗108\n氨氮92\n总磷131\n总磷海水147\n总氮76\n总氮海水92"
    n181 = Wait (ms)(milliseconds to wait=u32 1000 ("等待时间（毫秒）")) -> ()  [unwired: 1 out]
    n182 = global read "VAR氨氮全局变量.vi" "状态告警区"() -> (w340:T4)
    n183 = global read "氨氮断电保存全局变量.vi" "流程文件路径"() -> (w331:path)
    n184 = Bundle By Name(cluster=cluster{"命令":string, "data":variant} {"命令"="", "data"=variant} ("元素"), "命令"="读状态告警区", "data"=w342) -> (w351:cluster{"命令":string, "data":variant})
    n185 = local write "流程文件路径"(w331) -> ()
    n186 = Bundle By Name(cluster=cluster{"命令":string, "data":variant} {"命令"="", "data"=variant} ("元素"), "命令"="读测量数据区", "data"=w342) -> (w347:cluster{"命令":string, "data":variant})
    n187 = Unbundle By Name(w340) -> ("系统时间"=w339:timestamp)
    n188 = Enqueue Element(queue=w349, element=w351) -> (queue out=w345:refnum<queue>)  [unwired: 2 in, 2 out]
    n189 = Enqueue Element(queue=w345, element=w347) -> (queue out=w341:refnum<queue>)  [unwired: 2 in, 2 out]
    n190 = Get Date/Time In Seconds() -> (seconds since 1Jan1904=w338:timestamp)
    n191 = Subtract(x=w338, y=w339) -> (x-y=w337:dbl)
    n192 = Absolute Value(x=w337) -> (abs(x)=w336:dbl)
    n193 = global read "VAR氨氮全局变量.vi" "通讯状态"() -> (w332:bool)
    n194 = Greater Or Equal?(x=w336, y=120.0) -> (x >= y?=w334:bool)
    n195 = And(x=w332, y=w334) -> (x .and. y?=w333:bool)
    n196 = case shown="真" w333 {
      tunnel: w341 -> [_ w356]
      frame False {
      }
      frame True {
        n197 = call "氨氮启动命令.vi"("参数"=T5 {"站号"=3, "量程切换"=enum."AUTO", "控制命令"=enum."校时", "模式设置"=enum."待机", "测量间隔"=0}) -> ("启动命令"=w355:cluster{"命令":string, "data":variant})  [unwired: 10 in]
        n198 = Enqueue Element(queue=w356, element=w355) -> ()  [unwired: 2 in, 3 out]
      }
    }
    n199 = Increment(x=w344) -> (x+1=w343:enum16{"氨氮", "总磷"})
  }
  n200 = while {
    tunnel: w16 -> [w364]
    tunnel: w14 -> [w363]
    tunnel: w13 -> [w362]
    tunnel: w12 -> [w361]
    tunnel: w11 -> [w360]
    tunnel: w1 -> [w359]
    tunnel: w4 -> [w358]
    tunnel: w3 -> [_]
    stop <- FALSE stop-if-true
    n201 = event shown="[1] \"串口设置\": 值改变" {
      selector: _ -> [_ _ _ _ _ _ _ _ _ _ _ _ _ _ _ _ _ _ _]
      dyn-events: _ -> [_ _ _ _ _ _ _ _ _ _ _ _ _ _ _ _ _ _ _]
      timeout: _ -> [_ _ _ _ _ _ _ _ _ _ _ _ _ _ _ _ _ _ _]
      tunnel: w364 -> [_ w371 w400 _ _ _ _ _ w466 _ w491 w496 _ _ _ _ _ _ _]
      tunnel: w363 -> [_ _ _ _ _ _ _ _ _ _ _ _ _ _ _ w512 _ _ _]
      tunnel: w362 -> [_ _ _ _ _ _ _ _ _ _ _ _ _ _ _ w510 _ w528 w535]
      tunnel: w361 -> [_ _ _ _ _ _ _ _ _ _ _ _ _ _ _ w511 _ _ _]
      tunnel: w360 -> [_ _ _ _ _ _ _ _ _ _ _ _ _ _ _ w506 _ _ _]
      tunnel: w359 -> [_ _ _ _ _ _ _ _ _ _ _ _ _ _ _ _ _ w526 _]
      tunnel: w358 -> [_ _ _ _ _ _ _ _ _ _ _ w494 _ _ _ _ _ _ _]
      event Timeout {
        n202 = event-data() -> ()  [unwired: 1 in, 3 out]
      }
      event "串口设置": Value Change {
        n203 = event-data() -> ()  [unwired: 1 in, 6 out]
        n204 = global read "氨氮断电保存全局变量.vi" "VISA Resource"() -> (w374:refnum<visa-resource-name>)
        n205 = global read "氨氮断电保存全局变量.vi" "PORT"() -> (w369:string)
        n206 = global read "氨氮断电保存全局变量.vi" "IP"() -> (w370:string)
        n207 = call "串口配置.vi"("PORT"=w369, "IP"=w370, "请选择串口:"=w374) -> ("PORT 2"=w367:string, "IP 2"=w368:string, "确认 2"=w373:bool, "VISA资源名称 2"=w372:refnum<visa-resource-name>, "MB通信方式选择 2"=w366:enum16{"串口", "TCP"})  [unwired: 4 in]
        n208 = case shown="真" w373 {
          tunnel: w372 -> [_ w379]
          tunnel: w371 -> [_ w378]
          tunnel: w368 -> [_ w377]
          tunnel: w367 -> [_ w376]
          tunnel: w366 -> [_ w375]
          frame False {
          }
          frame True {
            n209 = flat-sequence {
              tunnel: w379 -> [w385]
              tunnel: w378 -> [w383]
              tunnel: w377 -> [w382]
              tunnel: w376 -> [w381]
              tunnel: w375 -> [w380]
              frame #0 {
                n210 = global write "氨氮断电保存全局变量.vi" "MB通信方式选择"(w380) -> ()
                n211 = global write "氨氮断电保存全局变量.vi" "VISA Resource"(w385) -> ()
                n212 = global write "氨氮断电保存全局变量.vi" "PORT"(w381) -> ()
                n213 = global write "氨氮断电保存全局变量.vi" "IP"(w382) -> ()
                n214 = Enqueue Element(queue=w383, element=cluster{"命令":string, "data":variant} {"命令"="启用模块", "data"=variant} ("元素")) -> ()  [unwired: 2 in, 3 out]
              }
              frame #1 {
                n215 = call <vilib>:"Application Directory.vi"() -> ("Application Directory"=w399:path)
                n216 = Build Path(base path=w399, name or relative path="data\\sys.ini" ("名称或相对路径")) -> (appended path=w397:path)
                n217 = call <vilib>:"Open Config Data.vi"("configuration file path"=w397) -> ("error out"=w393:errorcluster, "refnum"=w396:T13)  [unwired: 8 in, 1 out]
                n218 = vi-ref "氨氮断电保存全局变量.vi"() -> (w395:refnum<vi>)
                n219 = call <userlib>:"Write Panel to INI__ogtk.vi"("error in (no error)"=w393, "VI ref"=w395, "refnum"=w396) -> ("error out"=w392:errorcluster, "refnum out"=w394:T13)  [unwired: 7 in]
                n220 = call <vilib>:"Close Config Data.vi"("error in (no error)"=w392, "refnum"=w394) -> ("error out"=w387:errorcluster, "file path"=w386:path)  [unwired: 8 in]
                n221 = Open/Create/Replace File(file path (use dialog)=w386, error in=w387) -> (refnum out=w390:refnum<file>, error out=w391:errorcluster)  [unwired: 4 in, 1 out]
                n222 = Flush File(refnum=w390, error in=w391) -> (refnum out=w389:refnum<file>, error out=w388:errorcluster)
                n223 = Close File(refnum=w389, error in=w388) -> ()  [unwired: 2 out]
              }
            }
          }
        }
      }
      event "模块启用": Value Change {
        n224 = event-data() -> ("OldVal"=w401:bool)  [unwired: 1 in, 5 out]
        n225 = case shown="假" w401 {
          tunnel: w400 -> [w402 w404]
          frame False {
            n226 = Enqueue Element(queue=w402, element=cluster{"命令":string, "data":variant} {"命令"="停用模块", "data"=variant} ("元素")) -> ()  [unwired: 2 in, 3 out]
          }
          frame True {
            n227 = Enqueue Element(queue=w404, element=cluster{"命令":string, "data":variant} {"命令"="启用模块", "data"=variant} ("元素")) -> ()  [unwired: 2 in, 3 out]
          }
        }
      }
      event "流程文件路径": Value Change {
        n228 = event-data() -> ()  [unwired: 1 in, 6 out]
        n229 = flat-sequence {
          frame #0 {
            n230 = local read "流程文件路径"() -> (w406:path)
            n231 = global write "氨氮断电保存全局变量.vi" "流程文件路径"(w406) -> ()
          }
          frame #1 {
            n232 = call <vilib>:"Application Directory.vi"() -> ("Application Directory"=w420:path)
            n233 = Build Path(base path=w420, name or relative path="data\\sys.ini" ("名称或相对路径")) -> (appended path=w418:path)
            n234 = call <vilib>:"Open Config Data.vi"("configuration file path"=w418) -> ("error out"=w414:errorcluster, "refnum"=w417:T13)  [unwired: 8 in, 1 out]
            n235 = vi-ref "氨氮断电保存全局变量.vi"() -> (w416:refnum<vi>)
            n236 = call <userlib>:"Write Panel to INI__ogtk.vi"("error in (no error)"=w414, "VI ref"=w416, "refnum"=w417) -> ("error out"=w413:errorcluster, "refnum out"=w415:T13)  [unwired: 7 in]
            n237 = call <vilib>:"Close Config Data.vi"("error in (no error)"=w413, "refnum"=w415) -> ("error out"=w408:errorcluster, "file path"=w407:path)  [unwired: 8 in]
            n238 = Open/Create/Replace File(file path (use dialog)=w407, error in=w408) -> (refnum out=w411:refnum<file>, error out=w412:errorcluster)  [unwired: 4 in, 1 out]
            n239 = Flush File(refnum=w411, error in=w412) -> (refnum out=w410:refnum<file>, error out=w409:errorcluster)
            n240 = Close File(refnum=w410, error in=w409) -> ()  [unwired: 2 out]
          }
        }
      }
      event "公式一键写入": Value Change {
        n241 = event-data() -> ()  [unwired: 1 in, 6 out]
        n242 = local read "公式"() -> (w421:cluster{"X^2":dbl, "X":dbl, "b":dbl})
        n243 = call "公式复合写入.vi"("公式"=w421) -> ()  [unwired: 11 in]
      }
      event "曲线模型": Value Change {
        n244 = event-data() -> ()  [unwired: 1 in, 6 out]
        n245 = local write "公式"("曲线模型") -> ()
      }
      event "质控参数设置": Value Change {
        n246 = event-data() -> ()  [unwired: 1 in, 6 out]
        n247 = global read "氨氮断电保存全局变量.vi" "质控参数设置"() -> (w423:T19)
        n248 = call "质控参数设置.vi"("质控参数设置"=w423) -> ("输出簇"=w424:T20)  [unwired: 10 in]
        n249 = Unbundle By Name(w424) -> ("确定"=w425:bool)
        n250 = case shown="真" w425 {
          tunnel: w424 -> [_ w427]
          tunnel: w423 -> [_ w426]
          frame False {
          }
          frame True {
            n251 = flat-sequence {
              tunnel: w427 -> [w434]
              tunnel: w426 -> [w428]
              frame #0 {
                n252 = Unbundle By Name(w434) -> ("跨度值"=w433:dbl, "零点标准液浓度"=w432:dbl, "跨度标准液浓度"=w431:dbl, "标准液标准浓度"=w430:dbl)
                n253 = Bundle By Name(cluster=w428, "跨度值"=w433, "零点标准液浓度"=w432, "跨度标准液浓度"=w431, "标准液标准浓度"=w430) -> (w429:T19)
                n254 = global write "氨氮断电保存全局变量.vi" "质控参数设置"(w429) -> ()
              }
              frame #1 {
                n255 = call <vilib>:"Application Directory.vi"() -> ("Application Directory"=w435:path)
                n256 = Build Path(base path=w435, name or relative path="data\\sys.ini" ("名称或相对路径")) -> (appended path=w437:path)
                n257 = call <vilib>:"Open Config Data.vi"("configuration file path"=w437) -> ("error out"=w441:errorcluster, "refnum"=w438:T13)  [unwired: 8 in, 1 out]
                n258 = vi-ref "氨氮断电保存全局变量.vi"() -> (w439:refnum<vi>)
                n259 = call <userlib>:"Write Panel to INI__ogtk.vi"("error in (no error)"=w441, "VI ref"=w439, "refnum"=w438) -> ("error out"=w442:errorcluster, "refnum out"=w440:T13)  [unwired: 7 in]
                n260 = call <vilib>:"Close Config Data.vi"("error in (no error)"=w442, "refnum"=w440) -> ("error out"=w447:errorcluster, "file path"=w448:path)  [unwired: 8 in]
                n261 = Open/Create/Replace File(file path (use dialog)=w448, error in=w447) -> (refnum out=w444:refnum<file>, error out=w443:errorcluster)  [unwired: 4 in, 1 out]
                n262 = Flush File(refnum=w444, error in=w443) -> (refnum out=w445:refnum<file>, error out=w446:errorcluster)
                n263 = Close File(refnum=w445, error in=w446) -> ()  [unwired: 2 out]
              }
            }
          }
        }
      }
      event "氨氮自动测试量程配置": Value Change {
        n264 = event-data() -> ()  [unwired: 1 in, 6 out]
        n265 = flat-sequence {
          frame #0 {
            n266 = global write "氨氮断电保存全局变量.vi" "氨氮自动测试量程配置"("氨氮自动测试量程配置") -> ()
          }
          frame #1 {
            n267 = call <vilib>:"Application Directory.vi"() -> ("Application Directory"=w463:path)
            n268 = Build Path(base path=w463, name or relative path="data\\sys.ini" ("名称或相对路径")) -> (appended path=w461:path)
            n269 = call <vilib>:"Open Config Data.vi"("configuration file path"=w461) -> ("error out"=w457:errorcluster, "refnum"=w460:T13)  [unwired: 8 in, 1 out]
            n270 = vi-ref "氨氮断电保存全局变量.vi"() -> (w459:refnum<vi>)
            n271 = call <userlib>:"Write Panel to INI__ogtk.vi"("error in (no error)"=w457, "VI ref"=w459, "refnum"=w460) -> ("error out"=w456:errorcluster, "refnum out"=w458:T13)  [unwired: 7 in]
            n272 = call <vilib>:"Close Config Data.vi"("error in (no error)"=w456, "refnum"=w458) -> ("error out"=w451:errorcluster, "file path"=w450:path)  [unwired: 8 in]
            n273 = Open/Create/Replace File(file path (use dialog)=w450, error in=w451) -> (refnum out=w454:refnum<file>, error out=w455:errorcluster)  [unwired: 4 in, 1 out]
            n274 = Flush File(refnum=w454, error in=w455) -> (refnum out=w453:refnum<file>, error out=w452:errorcluster)
            n275 = Close File(refnum=w453, error in=w452) -> ()  [unwired: 2 out]
          }
        }
      }
      event "手动启动": Value Change {
        n276 = event-data() -> ()  [unwired: 1 in, 6 out]
        n277 = call "氨氮启动参数对话框.vi"() -> ("确认"=w464:bool, "元素"=w465:cluster{"命令":string, "data":variant})  [unwired: 10 in]
        n278 = case shown="真" w464 {
          tunnel: w466 -> [_ w468]
          tunnel: w465 -> [_ w467]
          frame False {
          }
          frame True {
            n279 = Enqueue Element(queue=w468, element=w467) -> ()  [unwired: 2 in, 3 out]
          }
        }
      }
      event "定时启动": Mouse Down {
        n280 = event-data() -> ()  [unwired: 1 in, 6 out]
        n281 = flat-sequence {
          frame #0 {
            n282 = global read "氨氮断电保存全局变量.vi" "定时控制"() -> (w469:T7)
            n283 = call "周期设置.vi"("定时控制参数输入"=w469) -> ("定时控制参数输出"=w470:T7)  [unwired: 10 in]
            n284 = global write "氨氮断电保存全局变量.vi" "定时控制"(w470) -> ()
          }
          frame #1 {
            n285 = call <vilib>:"Application Directory.vi"() -> ("Application Directory"=w484:path)
            n286 = Build Path(base path=w484, name or relative path="data\\sys.ini" ("名称或相对路径")) -> (appended path=w482:path)
            n287 = call <vilib>:"Open Config Data.vi"("configuration file path"=w482) -> ("error out"=w478:errorcluster, "refnum"=w481:T13)  [unwired: 8 in, 1 out]
            n288 = vi-ref "氨氮断电保存全局变量.vi"() -> (w480:refnum<vi>)
            n289 = call <userlib>:"Write Panel to INI__ogtk.vi"("error in (no error)"=w478, "VI ref"=w480, "refnum"=w481) -> ("error out"=w477:errorcluster, "refnum out"=w479:T13)  [unwired: 7 in]
            n290 = call <vilib>:"Close Config Data.vi"("error in (no error)"=w477, "refnum"=w479) -> ("error out"=w472:errorcluster, "file path"=w471:path)  [unwired: 8 in]
            n291 = Open/Create/Replace File(file path (use dialog)=w471, error in=w472) -> (refnum out=w475:refnum<file>, error out=w476:errorcluster)  [unwired: 4 in, 1 out]
            n292 = Flush File(refnum=w475, error in=w476) -> (refnum out=w474:refnum<file>, error out=w473:errorcluster)
            n293 = Close File(refnum=w474, error in=w473) -> ()  [unwired: 2 out]
          }
        }
      }
      event "单步测试": Value Change {
        w486 = u16 1 items=["总磷"=1, "氨氮"=3] ("站号")
        n294 = event-data() -> ()  [unwired: 1 in, 6 out]
        n295 = Bundle("站号"=w486, "总磷氨氮调试"="总磷氨氮调试") -> (w485:cluster{"站号":u16, "总磷氨氮调试":u16[]})  [unwired: 1 in]
        n296 = Bundle By Name(cluster=cluster{"命令":string, "data":variant} {"命令"="", "data"=variant} ("元素"), "命令"="debug", "data"=w485) -> (w488:cluster{"命令":string, "data":variant})
        n297 = Enqueue Element(queue=w491, element=w488) -> ()  [unwired: 2 in, 3 out]
      }
      event "停止": Value Change {
        n298 = event-data() -> ()  [unwired: 1 in, 6 out]
        n299 = Enqueue Element(queue=w496, element=cluster{"命令":string, "data":variant} {"命令"="启动", "data"=variant(cluster{"站号":u16, "控制命令输出":u16[]} {"站号"=3, "控制命令输出"=[2816]})} ("启动命令")) -> ()  [unwired: 2 in, 3 out]
        n300 = Cancel Notification(0:w494) -> (8:w493:refnum<notifier>)  [unwired: 1 in, 2 out]
        n301 = Send Notification(notification=TRUE ("通知"), notifier=w493) -> ()  [unwired: 1 in, 2 out]
      }
      event "设置": Value Change {
        n302 = event-data() -> ()  [unwired: 1 in, 6 out]
        n303 = property on="窗格" class="Pane"("Origin"=T10 {"Horizontal"=0, "Vertical"=628} ("原点")) -> ()  [unwired: 2 in, 2 out]
      }
      event "返回": Value Change {
        n304 = event-data() -> ()  [unwired: 1 in, 6 out]
        n305 = property on="窗格" class="Pane"("Origin"=T10 {"Horizontal"=0, "Vertical"=0} ("原点")) -> ()  [unwired: 2 in, 2 out]
      }
      event "公式.X^2", "公式.X", "公式.b": Mouse Down {
        n306 = event-data() -> ("CtlRef"=w502:refnum<vi>)  [unwired: 1 in, 5 out]
        n307 = property class="DigNum (严格)"(reference=w502) -> (reference out=w500:refnum<vi>, "Value"=w501:dbl)  [unwired: 1 in, 1 out]
        n308 = call "数字键盘.vi"("OldNumber"=w501) -> ("NewNumber"=w499:dbl)
        n309 = property class="DigNum (严格)"(reference=w500, "Val(Sgnl)"=w499) -> ()  [unwired: 1 in, 2 out]
      }
      event "读公式": Value Change {
        n310 = event-data() -> ()  [unwired: 1 in, 6 out]
        n311 = property class="Enum (严格)"(reference=w510) -> ("Value"=w509:enum16{"氨氮", "总磷"})  [unwired: 1 in, 2 out]
        n312 = property class="Enum (严格)"(reference=w511) -> ("Value"=w508:enum16{"水样测量", "空白核查", "跨度核查", "标样核查", "加标回收"})  [unwired: 1 in, 2 out]
        n313 = property class="Enum (严格)"(reference=w512) -> ("Value"=w507:enum16{"低量程", "高量程"})  [unwired: 1 in, 2 out]
        n314 = call "总磷氨氮公式读取_N.vi"("量程"=w507, "测量模式"=w508, "测量参数"=w509) -> ("error out"=w504:errorcluster, "公式"=w505:cluster{"X^2":dbl, "X":dbl, "b":dbl})  [unwired: 7 in]
        n315 = property class="Clust (严格)"(reference=w506, "Value"=w505) -> ()  [unwired: 1 in, 2 out]
        n316 = case shown="错误" w504 {
          tunnel: ["读取成功" ("消息") "读取失败" ("消息")] -> w503
          frame No Error {
          }
          frame Error {
          }
        }
        n317 = One Button Dialog(message=w503) -> ()  [unwired: 1 in, 1 out]
      }
      event "写公式": Value Change {
        n318 = event-data() -> ()  [unwired: 1 in, 6 out]
        n319 = call "总磷氨氮公式写入_N.vi"("公式"="公式", "量程"="量程下拉列表", "测量模式"="测量模式下拉列表", "测量参数"="参数下拉列表") -> ("error out"=w515:errorcluster)  [unwired: 7 in]
        n320 = case shown="无错误" w515 {
          tunnel: ["写入成功" ("消息") "写入失败" ("消息")] -> w516
          frame No Error {
          }
          frame Error {
          }
        }
        n321 = One Button Dialog(message=w516) -> ()  [unwired: 1 in, 1 out]
      }
      event "备用系数读取": Value Change {
        n322 = event-data() -> ()  [unwired: 1 in, 6 out]
        n323 = property class="Enum (严格)"(reference=w528) -> ("Value"=w527:enum16{"氨氮", "总磷"})  [unwired: 1 in, 2 out]
        n324 = call "总磷氨氮量程读取N.vi"("测量参数"=w527) -> ("error out"=w524:errorcluster, "量程参数读取"=w523:T1)  [unwired: 9 in]
        n325 = property class="Clust (严格)"(reference=w526, "Value"=w523) -> ()  [unwired: 1 in, 2 out]
        n326 = case shown="错误" w524 {
          tunnel: ["读取成功" ("消息") "读取失败" ("消息")] -> w525
          frame No Error {
          }
          frame Error {
          }
        }
        n327 = One Button Dialog(message=w525) -> ()  [unwired: 1 in, 1 out]
      }
      event "备用系数写入": Value Change {
        n328 = event-data() -> ()  [unwired: 1 in, 6 out]
        n329 = property class="Enum (严格)"(reference=w535) -> ("Value"=w534:enum16{"氨氮", "总磷"})  [unwired: 1 in, 2 out]
        n330 = call "总磷氨氮量程写入N.vi"("量程参数写入"="量程参数读取", "测量参数"=w534) -> ("error out"=w532:errorcluster)  [unwired: 8 in]
        n331 = case shown="无错误" w532 {
          tunnel: ["写入成功" ("消息") "写入失败" ("消息")] -> w533
          frame No Error {
          }
          frame Error {
          }
        }
        n332 = One Button Dialog(message=w533) -> ()  [unwired: 1 in, 1 out]
      }
    }
  }
